vi "forceQueue.vi"(8 "error in (no error)":errorcluster, 9 "Stop":bool, 10 "ByteArrayIn":u8[](array[numeric]), 11 "Command":T1) -> (0 "error out":errorcluster, 1 "Stop":bool, 2 "ByteArrayOut":u8[](array[numeric]))   [LabVIEW 2017, in "externalAquisition.lvlib"]
uses:
  externalAquisition.lvlib
  TypeDefs/QueueCommands.ctl
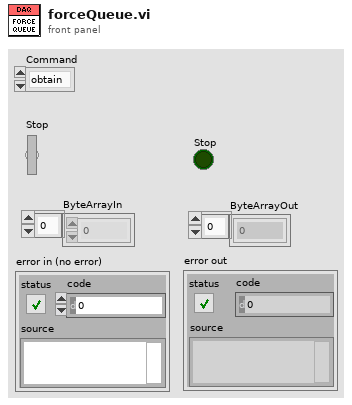
[diagram p1: front panel]
types:
  T1 = typedef "externalAquisition.lvlib/QueueCommands.ctl" = enum16{"obtain", "enqueue", "dequeue", "release"}
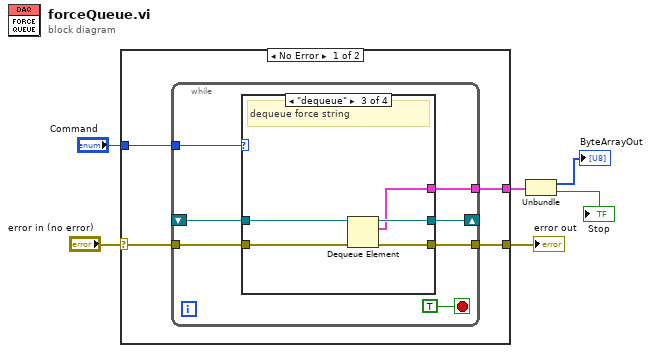
[diagram p0: block diagram]
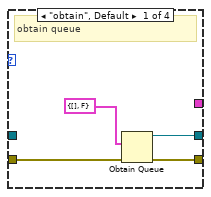
[diagram p2: hidden frame]
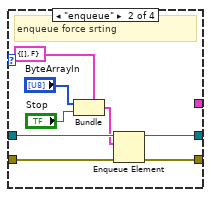
[diagram p3: hidden frame]
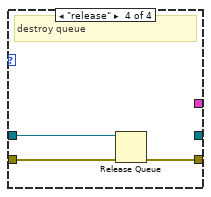
[diagram p4: hidden frame]
diagram:
  n1 = case shown="No Error" "error in (no error)" {
    selector: "error in (no error)" -> [w9 w38]
    tunnel: "Command" -> [w10 _]
    tunnel: [w8 w38] -> w4
    tunnel: [w7 _] -> w3
    frame No Error {
      n2 = while {
        tunnel: w10 -> [w16]
        tunnel: w9 -> [w15]
        tunnel: [w14] -> w8
        shift-right: [w13] -> _
        shift-left: _ -> [w12]
        tunnel: [w11] -> w7
        stop <- TRUE stop-if-true
        n3 = case shown="\"dequeue\"" w16 {
          tunnel: w15 -> [w21 w29 w32 w37]
          tunnel: [w20 w28 w31 w36] -> w14
          tunnel: [w19 w27 w34 _] -> w13
          tunnel: w12 -> [_ w26 w33 w35]
          tunnel: [_ _ w30 _] -> w11
          frame "obtain", Default {
            # "obtain queue"
            n4 = Obtain Queue(element data type=cluster{u8[], "Stop":bool} {[], "Stop"=FALSE}, error in (no error)=w21) -> (queue out=w19:refnum<queue>, error out=w20:errorcluster)  [unwired: 3 in, 1 out]
          }
          frame "enqueue" {
            # "enqueue force srting"
            n5 = Bundle(cluster=cluster{u8[], "Stop":bool} {[], "Stop"=FALSE}, "ByteArrayIn", "Stop"="Stop") -> (w22:cluster{u8[], "Stop":bool})
            n6 = Enqueue Element(queue=w26, element=w22, error in (no error)=w29) -> (queue out=w27:refnum<queue>, error out=w28:errorcluster)  [unwired: 1 in, 1 out]
          }
          frame "dequeue" {
            # "dequeue force string"
            n7 = Dequeue Element(queue=w33, error in (no error)=w32) -> (queue out=w34:refnum<queue>, element=w30:cluster{u8[], "Stop":bool}, error out=w31:errorcluster)  [unwired: 1 in, 1 out]
          }
          frame "release" {
            # "destroy queue"
            n8 = Release Queue(queue=w35, error in (no error)=w37) -> (error out=w36:errorcluster)  [unwired: 1 in, 2 out]
          }
        }
      }
    }
    frame Error {
    }
  }
  "error out" <- w4
  n9 = Unbundle(w3) -> (→"ByteArrayOut":u8[], "Stop"=→"Stop":bool)
